vi "lockin - Restore Saved AO.vi"(8 "error in (no error)":errorcluster, 11 "Instrument.DAQ":refnum<class "Instrument.DAQ.lvclass">) -> (0 "error out":errorcluster, 3 "Instrument.DAQ out":refnum<class "Instrument.DAQ.lvclass">)   [LabVIEW 2019, in "Instrument.DAQ.lvclass"]
uses:
  Instrument.DAQ.lvclass
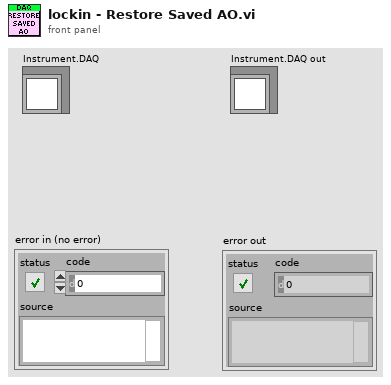
[diagram p1: front panel]
types:
  T1 = typedef "Instrument.DAQ.lvclass/AO.Channel--Cluster--Array.ctl" = T2[]
  T2 = typedef "Instrument.DAQ.lvclass/AO.Channel--Cluster.ctl" = cluster{"Enable?":bool, "Channel":i32, "Amplitude":dbl, "Offset":dbl, "Frequency":dbl, "Phase":dbl, "Function":T3, "Sweeping?":bool}
  T3 = typedef "Instrument.DAQ.lvclass/AO.Channel.Function--Enum.ctl" = enum16{"Sine", "Triangle", "Square"}
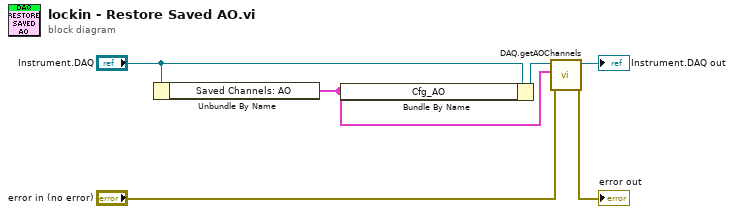
[diagram p0: block diagram]
diagram:
  n1 = Unbundle By Name("Instrument.DAQ") -> ("Saved Channels: AO"=w1:T1)
  n2 = Bundle By Name(cluster="Instrument.DAQ", "Cfg_AO"=w1) -> (w3:refnum<class "Instrument.DAQ.lvclass">)
  n3 = call "DAQ.getAOChannels.vi"("error in (no error)"="error in (no error)", "Channels: AO"=w1, "Instrument.DAQ"=w3) -> ("error out"=→"error out":errorcluster, "Instrument.DAQ out"=→"Instrument.DAQ out":refnum<class "Instrument.DAQ.lvclass">)  [unwired: 7 in]
